vi "Write RM DMA.vi"(8 "error in":errorcluster, 9 "VMIC reference in":T2, 10 "Block descriptors":T1[](array[typedef]), 11 "Values":dbl[](array[numeric])) -> (0 "error out":errorcluster, 1 "VMIC reference out":T2, 2 "Write Duration":u32, 3 "Values":dbl[](array[numeric]))   [LabVIEW 2017, in "GE_RM_Real Time.lvlib"]
uses:
  GE_RM_Real Time.lvlib
  Shared/Block descriptor.ctl
  Shared/GE_RM_Shared.lvlib
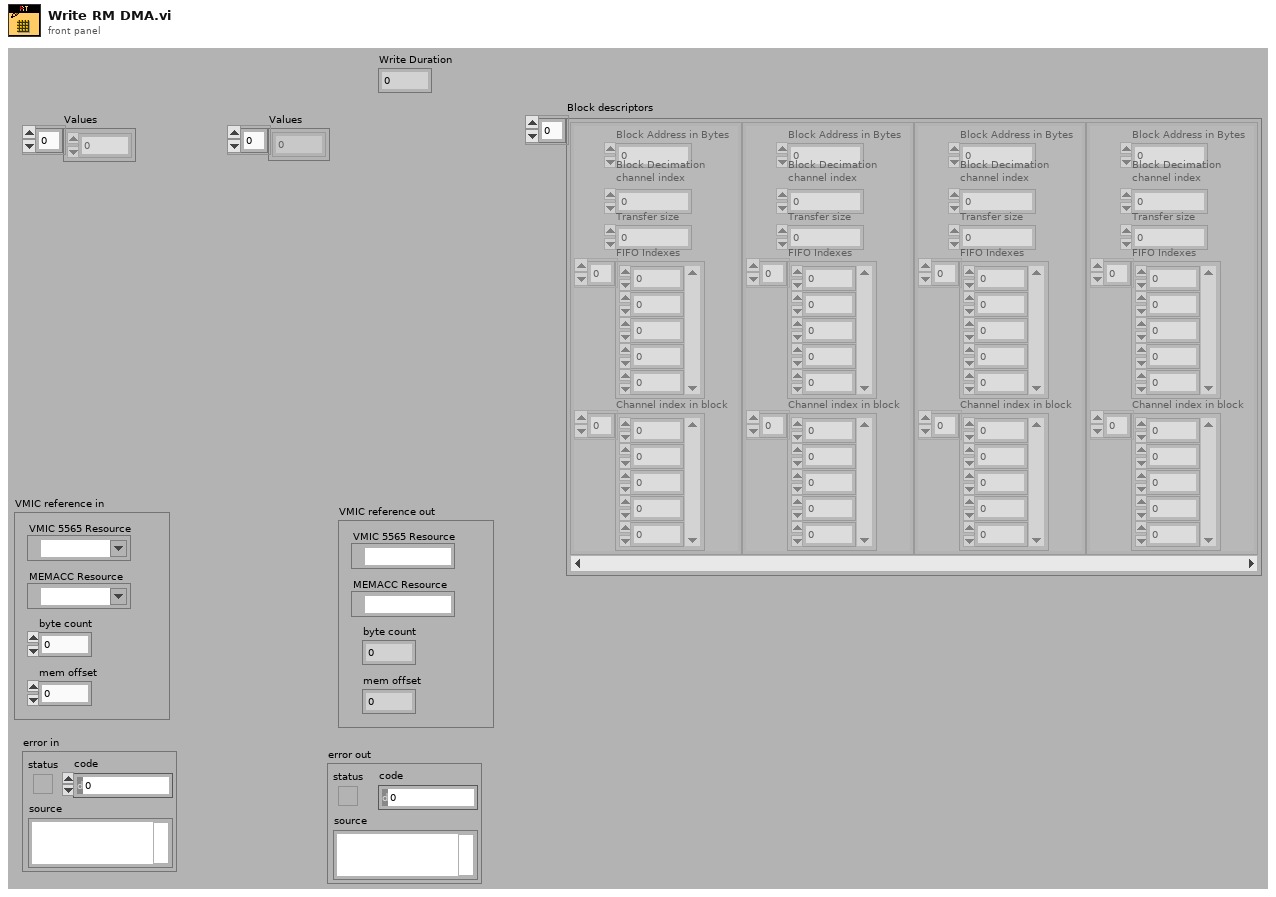
[diagram p1: front panel]
types:
  T1 = typedef "GE_RM_Shared.lvlib/Block descriptor.ctl" = cluster{"Block Address in Bytes":u32, "Block Decimation \nchannel index":i32, "Transfer size":u32, "FIFO Indexes":i32[], "Channel index in block":i32[]}
  T2 = cluster{"VMIC 5565 Resource":refnum<visa-resource-name>, "MEMACC Resource":refnum<visa-resource-name>, "byte count":u32, "mem offset":u32}
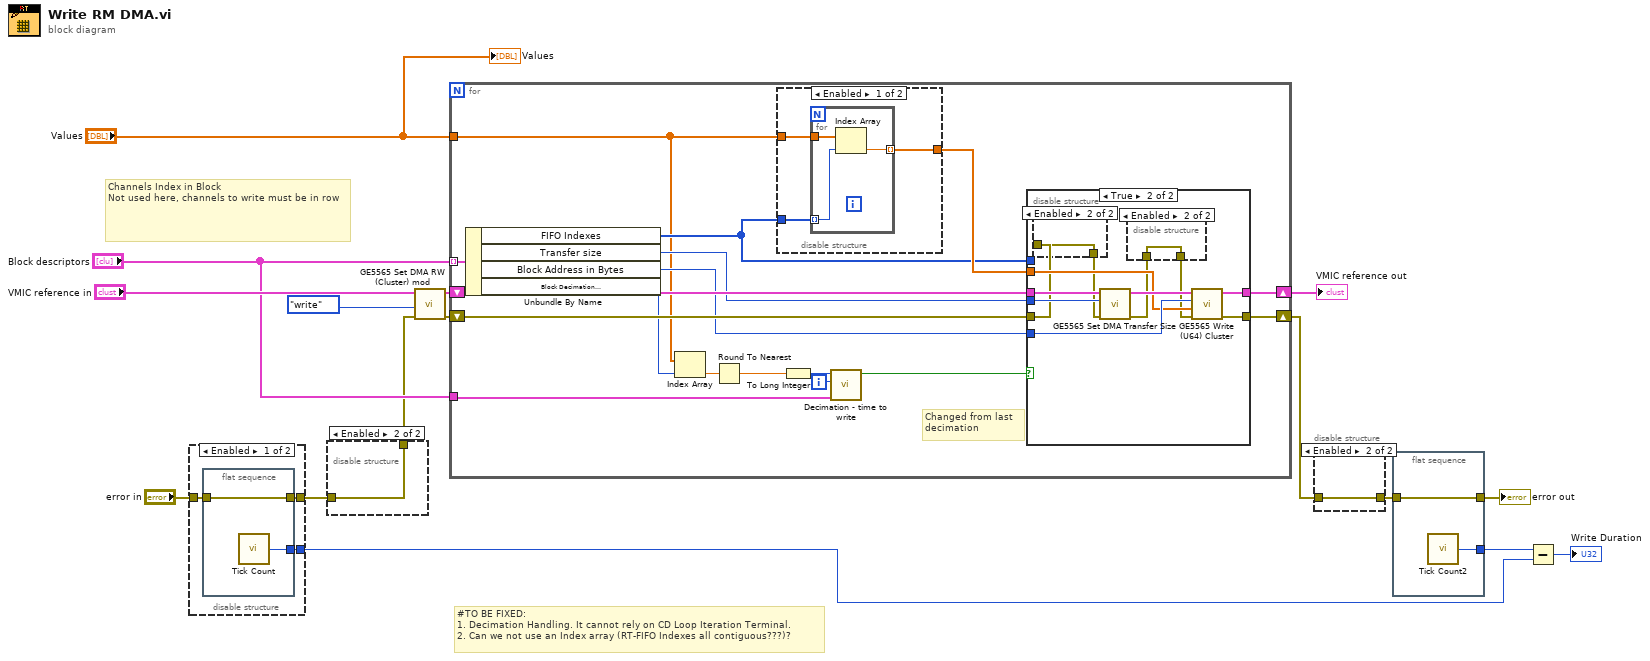
[diagram p0: block diagram]
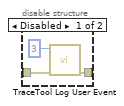
[diagram p2: hidden frame]
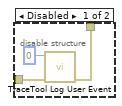
[diagram p3: hidden frame]
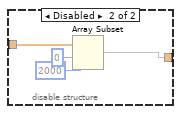
[diagram p4: hidden frame]
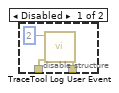
[diagram p6: hidden frame]
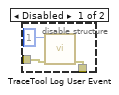
[diagram p7: hidden frame]
diagram:
  # "#TO BE FIXED:\n1. Decimation Handling. It cannot rely on CD Loop Iteration Terminal.\n2. Can we not use an Index array (RT-FIFO Indexes all contiguous???)?"
  # "Channels Index in Block\nNot used here, channels to write must be in row"
  n1 = disable-structure shown="Enabled" {
    disable-tunnel: "error in" -> [w19 w22]
    disable-tunnel: [w18 _] -> w6
    disable-tunnel: [w17 w22] -> w4
    frame Enabled {
      n2 = flat-sequence {
        tunnel: [w21] -> w17
        tunnel: w19 -> [w21]
        tunnel: [w20] -> w18
        frame #0 {
          n3 = call "Tick Count"() -> ("Tick Count(uSec)"=w20:u32)
        }
      }
    }
    frame Disabled {
    }
  }
  n4 = disable-structure shown="Enabled" {
    disable-tunnel: w4 -> [w25 w26]
    disable-tunnel: [w24 w26] -> w3
    frame Disabled {
      n5 = call <vilib>:"TraceTool Log User Event.vi"("error in (no error)"=w25, "Event ID (0-255)"=u32 0) -> ("error out"=w24:errorcluster)  [unwired: 9 in]
    }
    frame Enabled {
    }
  }
  n6 = call "GE5565 Set DMA RW (Cluster) mod.vi"("error in (no error)"=w3, "operation (read)"=enum16{"read", "write"}."write", "VMIC-5565"="VMIC reference in") -> ("error out"=w8:errorcluster, "VMIC-5565"=w9:T2)  [unwired: 3 in]
  n7 = for "Write Output Values to System" {
    shift-right: [w41] -> w2
    shift-left: w8 -> [w40]
    tunnel: "Values" -> [w34]
    shift-right: [w43] -> w7
    shift-left: w9 -> [w42]
    tunnel: "Block descriptors" -> [w39] mode=indexing
    tunnel: "Block descriptors" -> [w28]
    i -> [w27]
    # "Changed from last\ndecimation"
    n8 = Unbundle By Name(w39) -> ("FIFO Indexes"=w35:i32[], "Transfer size"=w37:u32, "Block Address in Bytes"=w38:u32, "Block Decimation \nchannel index"=w33:i32)
    n9 = Index Array(array=w34, index=w33) -> (element=w32:dbl)
    n10 = Round To Nearest(number=w32) -> (nearest integer value=w31:dbl)
    n11 = disable-structure shown="Enabled" {
      disable-tunnel: [w46 w50] -> w36
      disable-tunnel: w35 -> [w45 _]
      disable-tunnel: w34 -> [w44 w53]
      frame Enabled {
        n12 = for {
          tunnel: w45 -> [w47] mode=indexing
          tunnel: w44 -> [w49]
          tunnel: [w48] -> w46 mode=indexing
          n13 = Index Array(array=w49, index=w47) -> (element=w48:dbl)
        }
      }
      frame Disabled {
        n14 = Array Subset(array=w53, index=0, length=2000) -> (w50:dbl[])
      }
    }
    n15 = To Long Integer(number=w31) -> (32bit integer=w30:i32)
    n16 = call "Decimation - time to write.vi"("Block descriptors"=w28, "Iteration"=w27, "Decimation"=w30) -> ("Trigger?"=w29:bool)  [unwired: 8 in]
    n17 = case shown="True" w29 {
      tunnel: [w54 w66] -> w41
      tunnel: [w55 w65] -> w43
      tunnel: w40 -> [w54 w59]
      tunnel: w42 -> [w55 w64]
      tunnel: w37 -> [_ w63]
      tunnel: w38 -> [_ w62]
      tunnel: w36 -> [_ w60]
      tunnel: w35 -> [_ _]
      frame False {
      }
      frame True {
        n18 = disable-structure shown="Enabled" {
          disable-tunnel: w59 -> [w72 w74]
          disable-tunnel: [w71 w74] -> w58
          frame Disabled {
            n19 = call <vilib>:"TraceTool Log User Event.vi"("error in (no error)"=w72, "Event ID (0-255)"=u32 1) -> ("error out"=w71:errorcluster)  [unwired: 9 in]
          }
          frame Enabled {
          }
        }
        n20 = call "GE5565 Set DMA Transfer Size.vi"("error in (no error)"=w58, "Transfer Size"=w63, "VMIC-5565"=w64) -> ("error out"=w57:errorcluster, "VMIC-5565"=w61:T2)  [unwired: 3 in]
        n21 = disable-structure shown="Enabled" {
          disable-tunnel: w57 -> [w68 w70]
          disable-tunnel: [w67 w70] -> w56
          frame Disabled {
            n22 = call <vilib>:"TraceTool Log User Event.vi"("error in (no error)"=w68, "Event ID (0-255)"=u32 2) -> ("error out"=w67:errorcluster)  [unwired: 9 in]
          }
          frame Enabled {
          }
        }
        n23 = call "GE5565 Write (U64) Cluster.vi"("error in (no error)"=w56, "buffer"=w60, "offset (0)"=w62, "VMIC reference in"=w61) -> ("error out"=w66:errorcluster, "VMIC reference out"=w65:T2)  [unwired: 6 in]
      }
    }
  }
  "VMIC reference out" <- w7
  n24 = disable-structure shown="Enabled" {
    disable-tunnel: w2 -> [w76 w78]
    disable-tunnel: [w75 w78] -> w1
    frame Disabled {
      n25 = call <vilib>:"TraceTool Log User Event.vi"("error in (no error)"=w76, "Event ID (0-255)"=u32 3) -> ("error out"=w75:errorcluster)  [unwired: 9 in]
    }
    frame Enabled {
    }
  }
  n26 = flat-sequence {
    tunnel: [w80] -> w15
    tunnel: w1 -> [w80]
    tunnel: [w79] -> w14
    frame #0 {
      n27 = call "Tick Count2"() -> ("Tick Count(uSec)"=w79:u32)
    }
  }
  n28 = Subtract(x=w14, y=w6) -> (x-y=→"Write Duration":u32)
  "Values" <- "Values"
  "error out" <- w15
